vi "pumonarytesting_auto_attempt3.vi"() -> ()   [LabVIEW 2014]
uses:
  <vilib>/vision/NI_Vision_Development_Module.lvlib
  <instrlib>/KD Scientific 2XX Series/KD Scientific 2XX Series.lvlib
panel:
  in  "Number of Cycles":i32
  in  "Min Pressure":dbl
  in  "Max Pressure":dbl
  out "Status":T1
  in  "stop 2":bool
  out "Delivered Volume":dbl
  out "Units":string
  in  "Baud Rate (9600)":u32(ring)=9600 items=["300"=300, "1200"=1200, "2400"=2400, "4800"=4800, "9600"=9600]
  in  "Withdrawal Settings":T2={"Flow Rate (5)"=5.0, "Volume (10)"=10.0, "Volume Units (ml)"=enum."milliliters (ml)", "Rate Units (ml/min.)"=enum."milliliters per minute (ml/min.)"} {"Volume (10)" format="%#.3g"}
  in  "Diameter (8.75 mm)":dbl=8.75
  in  "Infusion Settings":T2={"Flow Rate (5)"=5.0, "Volume (10)"=10.0, "Volume Units (ml)"=enum."milliliters (ml)", "Rate Units (ml/min.)"=enum."milliliters per minute (ml/min.)"}
  in  "Address (0)":i32 format="%0.0f"
  in  "error in (no error)":errorcluster
  in  "VISA resource name":refnum<visa-resource-name>="COM1"
  in  "stop":bool
  out "Image":T3(plugin-control)
  out "Particle Measurements (Pixels) (Particle Analysis 1)":dbl[][](array[numeric]) format="%.2f"
  out "subarray":dbl[](array[numeric])
  out "The diameter":dbl[](array[numeric])
  in  "stop (F)":bool
  out "Data from Transducer":dynamicdata(graph) caption="Voltage from Transducer V"
  out "Voltage from pressure transducer":dbl[](array[numeric])
  out "Pressure mm Hg":dbl[](graph)
  in  "Calibration factor(-25.53)":dbl[](array[numeric])
  in  "Zero Error (-.09)":dbl[](array[numeric])
  out "pressure mm Hg":dbl[](array[numeric])
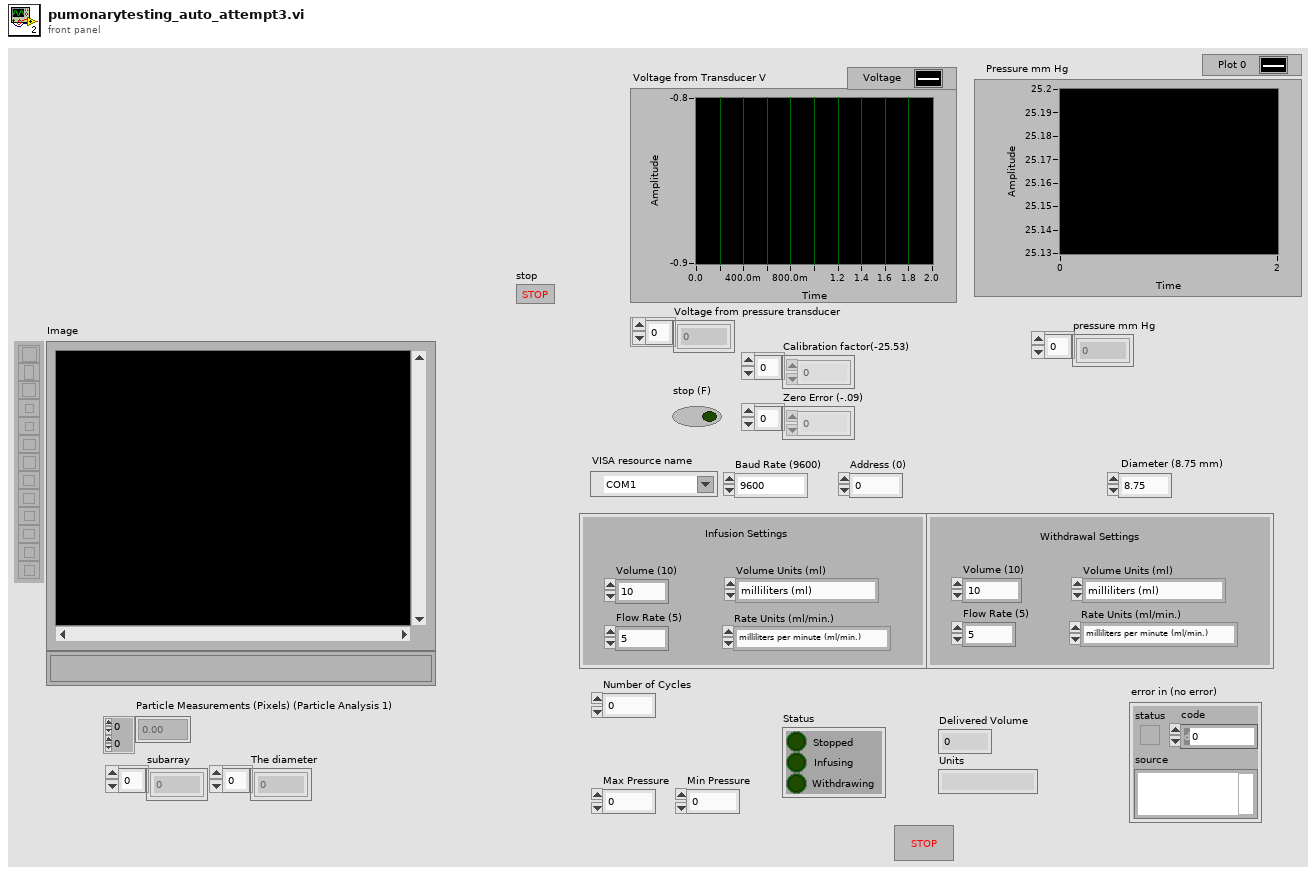
[diagram p1: front panel]
types:
  T1 = cluster{"Stopped":bool, "Infusing":bool, "Withdrawing":bool}
  T2 = cluster{"Flow Rate (5)":dbl, "Volume (10)":dbl, "Volume Units (ml)":enum16{"milliliters (ml)", "microliters (ul)"}, "Rate Units (ml/min.)":enum16{"milliliters per minute (ml/min.)", "milliliters per hour (ml/hr.)", "microliters per minute (ul/min.)", "microliters per hour (ul/hr.)"}}
  T3 = typedef "IMAQ Image.ctl" = refnum<image>
  T4 = typedef "Board Id" = u8
  T5 = typedef "ROI Descriptor" = cluster{"Global Rectangle":i32[], "Contours":cluster{"ID":enum32{"External", "Internal"}, "Type":u32, "Coordinates":i32[]}[]}
  T6 = enum16{"milliliters per minute (ml/min.)", "milliliters per hour (ml/hr.)", "microliters per minute (ul/min.)", "microliters per hour (ul/hr.)"}
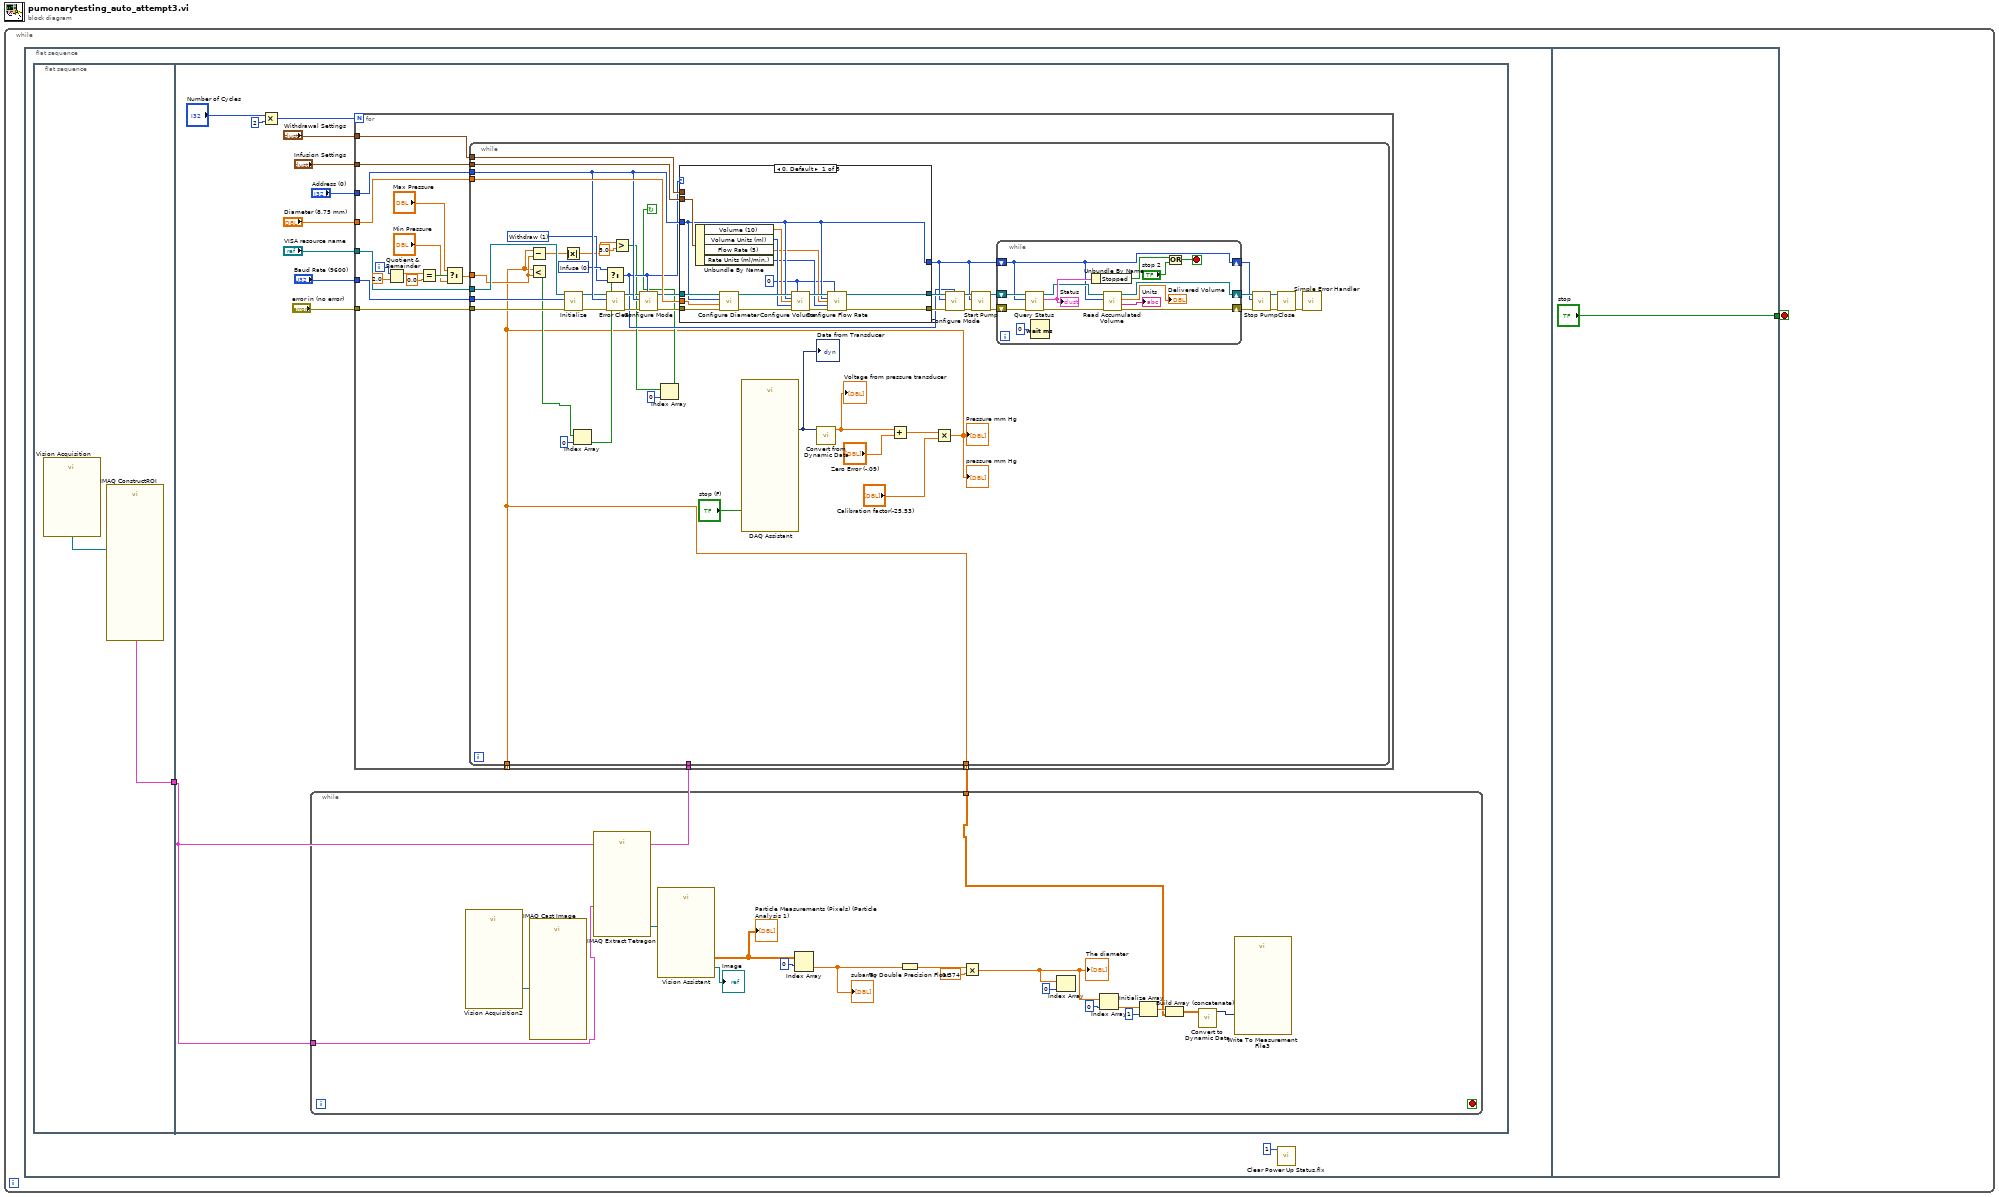
[diagram p0: block diagram]
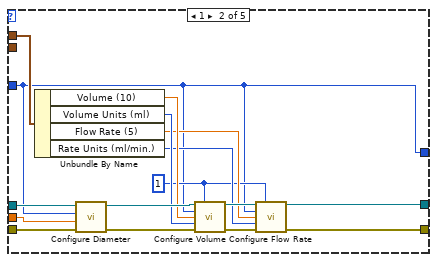
[diagram p2: hidden frame]
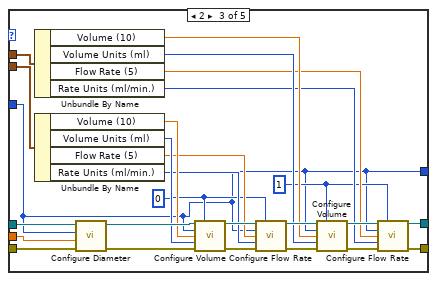
[diagram p3: hidden frame]
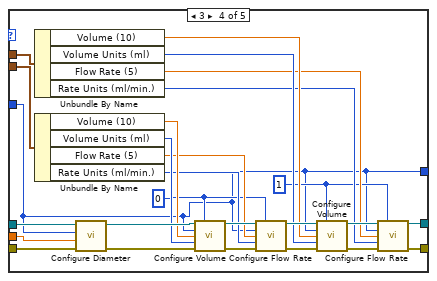
[diagram p4: hidden frame]
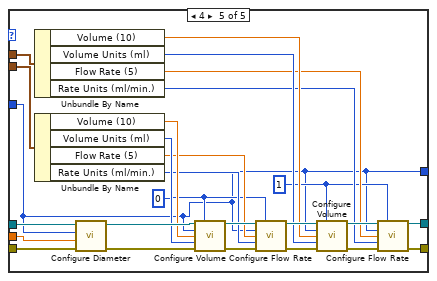
[diagram p5: hidden frame]
diagram:
  n1 = while {
    stop <- w1 stop-if-true
    n2 = flat-sequence {
      tunnel: ["stop"] -> w1
      frame #0 {
        n3 = flat-sequence {
          tunnel: [w4] -> w3
          tunnel: w3 -> [w6]
          frame #0 {
            n4 = call "Vision Acquisition"() -> ("Image Out"=w5:T3)  [unwired: 26 in, 1 out]
            n5 = call "IMAQ ConstructROI"("Image"=w5) -> ("ROI Descriptor Out"=w4:T5)  [unwired: 7 in, 3 out]
          }
          frame #1 {
            n6 = Multiply(x="Number of Cycles", y=2) -> (x*y=w17:i32)
            n7 = for {
              N: w17 -> [_]
              tunnel: "VISA resource name" -> [w53]
              tunnel: "error in (no error)" -> [w52]
              tunnel: "Infusion Settings" -> [w51]
              tunnel: "Withdrawal Settings" -> [w50]
              tunnel: "Diameter (8.75 mm)" -> [w49]
              tunnel: "Baud Rate (9600)" -> [w48]
              tunnel: "Address (0)" -> [w47]
              tunnel: [w38] -> _ mode=indexing
              tunnel: w6 -> [w37]
              tunnel: [w36] -> w7 mode=indexing
              i -> [w45]
              n8 = Quotient & Remainder(x=w45, y=2.0) -> (x-y*floor(x/y)=w43:dbl)  [unwired: 1 out]
              n9 = Equal?(x=w43, y=0.0) -> (x = y?=w42:bool)
              n10 = Select(t="Max Pressure", s=w42, f="Min Pressure") -> (s? t:f=w39:dbl)
              n11 = while {
                tunnel: w53 -> [w99]
                tunnel: w52 -> [w98]
                tunnel: w51 -> [w97]
                tunnel: w50 -> [w96]
                tunnel: w49 -> [w95]
                tunnel: w48 -> [w94]
                tunnel: w47 -> [w93]
                tunnel: w39 -> [w70]
                tunnel: [w54] -> w38
                tunnel: w37 -> [_]
                tunnel: [w54] -> w36
                stop <- w55 continue-if-true
                w72 = u16 1 items=["Withdraw"=1]
                w73 = u16 0 items=["Infuse"] ("Mode (infuse)")
                n12 = call <instrlib>:"Initialize.vi"("error in (no error)"=w98, "Baud Rate (9600)"=w94, "VISA resource name"=w99) -> ("error out"=w75:errorcluster, "VISA resource name out"=w74:refnum<visa-resource-name>)  [unwired: 7 in]
                n13 = call <instrlib>:"Error Clear.vi"("error in (no error)"=w75, "Address (0)"=w93, "VISA resource name"=w74) -> ("error out"=w76:errorcluster, "VISA resource name out"=w77:refnum<visa-resource-name>)  [unwired: 6 in, 1 out]
                n14 = call "DAQ Assistant"("stop (F)"="stop (F)") -> ("data"=w61:dynamicdata)  [unwired: 15 in, 3 out]
                "Data from Transducer" <- w61
                n15 = call "Convert from Dynamic Data"("Dynamic Data Type"=w61) -> ("Array"=w64:dbl[])  [unwired: 3 in]
                "Voltage from pressure transducer" <- w64
                n16 = Add(x=w64, y="Zero Error (-.09)") -> (x+y=w62:dbl[])
                n17 = Multiply(x=w62, y="Calibration factor(-25.53)") -> (x*y=w54:dbl[])
                "Pressure mm Hg" <- w54
                "pressure mm Hg" <- w54
                n18 = Subtract(x=w54, y=w70) -> (x-y=w69:dbl[])
                n19 = Less?(x=w54, y=w70) -> (x < y?=w60:bool[])
                n20 = Absolute Value(x=w69) -> (abs(x)=w68:dbl[])
                n21 = Index Array(array=w60, index=0) -> (element=w58:bool)
                n22 = Select(t=w73, s=w58, f=w72) -> (s? t:f=w71:u16)
                n23 = Greater?(x=w68, y=5.0) -> (0:w57:bool[])
                n24 = call <instrlib>:"Configure Mode.vi"("Mode (infuse)"=w71, "error in (no error)"=w76, "Address (0)"=w93, "VISA resource name"=w77) -> ("error out"=w79:errorcluster, "VISA resource name out"=w78:refnum<visa-resource-name>)  [unwired: 6 in]
                n25 = Index Array(array=w57, index=0) -> (element=w55:bool)
                n26 = case shown="0, Default" w71 {
                  tunnel: w97 -> [w109 _ w157 w183 w209]
                  tunnel: w96 -> [_ w131 w156 w182 w208]
                  tunnel: w78 -> [w115 w130 w155 w181 w207]
                  tunnel: w79 -> [w114 w126 w154 w180 w206]
                  tunnel: w95 -> [w108 w122 w137 w163 w189]
                  tunnel: [w107 w116 w132 w158 w184] -> w80
                  tunnel: w93 -> [w107 w116 w132 w158 w184]
                  tunnel: [w102 w127 w134 w160 w186] -> w84
                  tunnel: [w101 w123 w133 w159 w185] -> w83
                  frame 0, Default {
                    w100 = 0
                    n27 = Unbundle By Name(w109) -> ("Volume (10)"=w106:dbl, "Volume Units (ml)"=w105:enum16{"milliliters (ml)", "microliters (ul)"}, "Flow Rate (5)"=w104:dbl, "Rate Units (ml/min.)"=w103:T6)
                    n28 = call <instrlib>:"Configure Diameter.vi"("error in (no error)"=w114, "Diameter (8.75 mm)"=w108, "Address (0)"=w107, "VISA resource name"=w115) -> ("error out"=w112:errorcluster, "VISA resource name out"=w113:refnum<visa-resource-name>)  [unwired: 6 in]
                    n29 = call <instrlib>:"Configure Volume.vi"("VISA resource name"=w113, "Mode (infuse)"=w100, "Address (0)"=w107, "Volume (100)"=w106, "Units (0: milliliters)"=w105, "error in (no error)"=w112) -> ("VISA resource name out"=w111:refnum<visa-resource-name>, "error out"=w110:errorcluster)  [unwired: 8 in]
                    n30 = call <instrlib>:"Configure Flow Rate.vi"("VISA resource name"=w111, "Mode (infuse)"=w100, "Address (0)"=w107, "Flow Rate (5)"=w104, "Units (0: milliliters per minute)"=w103, "error in (no error)"=w110) -> ("VISA resource name out"=w102:refnum<visa-resource-name>, "error out"=w101:errorcluster)  [unwired: 8 in]
                  }
                  frame 1 {
                    w117 = 1
                    n31 = Unbundle By Name(w131) -> ("Volume (10)"=w121:dbl, "Volume Units (ml)"=w120:enum16{"milliliters (ml)", "microliters (ul)"}, "Flow Rate (5)"=w119:dbl, "Rate Units (ml/min.)"=w118:T6)
                    n32 = call <instrlib>:"Configure Diameter.vi"("error in (no error)"=w126, "Diameter (8.75 mm)"=w122, "Address (0)"=w116, "VISA resource name"=w130) -> ("error out"=w125:errorcluster, "VISA resource name out"=w129:refnum<visa-resource-name>)  [unwired: 6 in]
                    n33 = call <instrlib>:"Configure Volume.vi"("VISA resource name"=w129, "Mode (infuse)"=w117, "Address (0)"=w116, "Volume (100)"=w121, "Units (0: milliliters)"=w120, "error in (no error)"=w125) -> ("VISA resource name out"=w128:refnum<visa-resource-name>, "error out"=w124:errorcluster)  [unwired: 8 in]
                    n34 = call <instrlib>:"Configure Flow Rate.vi"("VISA resource name"=w128, "Mode (infuse)"=w117, "Address (0)"=w116, "Flow Rate (5)"=w119, "Units (0: milliliters per minute)"=w118, "error in (no error)"=w124) -> ("VISA resource name out"=w127:refnum<visa-resource-name>, "error out"=w123:errorcluster)  [unwired: 8 in]
                  }
                  frame 2 {
                    w135 = 1
                    w136 = 0
                    n35 = Unbundle By Name(w156) -> ("Volume (10)"=w141:dbl, "Volume Units (ml)"=w140:enum16{"milliliters (ml)", "microliters (ul)"}, "Flow Rate (5)"=w139:dbl, "Rate Units (ml/min.)"=w138:T6)
                    n36 = Unbundle By Name(w157) -> ("Volume (10)"=w145:dbl, "Volume Units (ml)"=w144:enum16{"milliliters (ml)", "microliters (ul)"}, "Flow Rate (5)"=w143:dbl, "Rate Units (ml/min.)"=w142:T6)
                    n37 = call <instrlib>:"Configure Diameter.vi"("error in (no error)"=w154, "Diameter (8.75 mm)"=w137, "Address (0)"=w132, "VISA resource name"=w155) -> ("error out"=w149:errorcluster, "VISA resource name out"=w153:refnum<visa-resource-name>)  [unwired: 6 in]
                    n38 = call <instrlib>:"Configure Volume.vi"("VISA resource name"=w153, "Mode (infuse)"=w136, "Address (0)"=w132, "Volume (100)"=w145, "Units (0: milliliters)"=w144, "error in (no error)"=w149) -> ("VISA resource name out"=w152:refnum<visa-resource-name>, "error out"=w148:errorcluster)  [unwired: 8 in]
                    n39 = call <instrlib>:"Configure Flow Rate.vi"("VISA resource name"=w152, "Mode (infuse)"=w136, "Address (0)"=w132, "Flow Rate (5)"=w143, "Units (0: milliliters per minute)"=w142, "error in (no error)"=w148) -> ("VISA resource name out"=w151:refnum<visa-resource-name>, "error out"=w147:errorcluster)  [unwired: 8 in]
                    n40 = call <instrlib>:"Configure Volume.vi"("VISA resource name"=w151, "Mode (infuse)"=w135, "Address (0)"=w132, "Volume (100)"=w141, "Units (0: milliliters)"=w140, "error in (no error)"=w147) -> ("VISA resource name out"=w150:refnum<visa-resource-name>, "error out"=w146:errorcluster)  [unwired: 8 in]
                    n41 = call <instrlib>:"Configure Flow Rate.vi"("VISA resource name"=w150, "Mode (infuse)"=w135, "Address (0)"=w132, "Flow Rate (5)"=w139, "Units (0: milliliters per minute)"=w138, "error in (no error)"=w146) -> ("VISA resource name out"=w134:refnum<visa-resource-name>, "error out"=w133:errorcluster)  [unwired: 8 in]
                  }
                  frame 3 {
                    w161 = 1
                    w162 = 0
                    n42 = Unbundle By Name(w182) -> ("Volume (10)"=w167:dbl, "Volume Units (ml)"=w166:enum16{"milliliters (ml)", "microliters (ul)"}, "Flow Rate (5)"=w165:dbl, "Rate Units (ml/min.)"=w164:T6)
                    n43 = Unbundle By Name(w183) -> ("Volume (10)"=w171:dbl, "Volume Units (ml)"=w170:enum16{"milliliters (ml)", "microliters (ul)"}, "Flow Rate (5)"=w169:dbl, "Rate Units (ml/min.)"=w168:T6)
                    n44 = call <instrlib>:"Configure Diameter.vi"("error in (no error)"=w180, "Diameter (8.75 mm)"=w163, "Address (0)"=w158, "VISA resource name"=w181) -> ("error out"=w175:errorcluster, "VISA resource name out"=w179:refnum<visa-resource-name>)  [unwired: 6 in]
                    n45 = call <instrlib>:"Configure Volume.vi"("VISA resource name"=w179, "Mode (infuse)"=w162, "Address (0)"=w158, "Volume (100)"=w171, "Units (0: milliliters)"=w170, "error in (no error)"=w175) -> ("VISA resource name out"=w178:refnum<visa-resource-name>, "error out"=w174:errorcluster)  [unwired: 8 in]
                    n46 = call <instrlib>:"Configure Flow Rate.vi"("VISA resource name"=w178, "Mode (infuse)"=w162, "Address (0)"=w158, "Flow Rate (5)"=w169, "Units (0: milliliters per minute)"=w168, "error in (no error)"=w174) -> ("VISA resource name out"=w177:refnum<visa-resource-name>, "error out"=w173:errorcluster)  [unwired: 8 in]
                    n47 = call <instrlib>:"Configure Volume.vi"("VISA resource name"=w177, "Mode (infuse)"=w161, "Address (0)"=w158, "Volume (100)"=w167, "Units (0: milliliters)"=w166, "error in (no error)"=w173) -> ("VISA resource name out"=w176:refnum<visa-resource-name>, "error out"=w172:errorcluster)  [unwired: 8 in]
                    n48 = call <instrlib>:"Configure Flow Rate.vi"("VISA resource name"=w176, "Mode (infuse)"=w161, "Address (0)"=w158, "Flow Rate (5)"=w165, "Units (0: milliliters per minute)"=w164, "error in (no error)"=w172) -> ("VISA resource name out"=w160:refnum<visa-resource-name>, "error out"=w159:errorcluster)  [unwired: 8 in]
                  }
                  frame 4 {
                    w187 = 1
                    w188 = 0
                    n49 = Unbundle By Name(w208) -> ("Volume (10)"=w193:dbl, "Volume Units (ml)"=w192:enum16{"milliliters (ml)", "microliters (ul)"}, "Flow Rate (5)"=w191:dbl, "Rate Units (ml/min.)"=w190:T6)
                    n50 = Unbundle By Name(w209) -> ("Volume (10)"=w197:dbl, "Volume Units (ml)"=w196:enum16{"milliliters (ml)", "microliters (ul)"}, "Flow Rate (5)"=w195:dbl, "Rate Units (ml/min.)"=w194:T6)
                    n51 = call <instrlib>:"Configure Diameter.vi"("error in (no error)"=w206, "Diameter (8.75 mm)"=w189, "Address (0)"=w184, "VISA resource name"=w207) -> ("error out"=w201:errorcluster, "VISA resource name out"=w205:refnum<visa-resource-name>)  [unwired: 6 in]
                    n52 = call <instrlib>:"Configure Volume.vi"("VISA resource name"=w205, "Mode (infuse)"=w188, "Address (0)"=w184, "Volume (100)"=w197, "Units (0: milliliters)"=w196, "error in (no error)"=w201) -> ("VISA resource name out"=w204:refnum<visa-resource-name>, "error out"=w200:errorcluster)  [unwired: 8 in]
                    n53 = call <instrlib>:"Configure Flow Rate.vi"("VISA resource name"=w204, "Mode (infuse)"=w188, "Address (0)"=w184, "Flow Rate (5)"=w195, "Units (0: milliliters per minute)"=w194, "error in (no error)"=w200) -> ("VISA resource name out"=w203:refnum<visa-resource-name>, "error out"=w199:errorcluster)  [unwired: 8 in]
                    n54 = call <instrlib>:"Configure Volume.vi"("VISA resource name"=w203, "Mode (infuse)"=w187, "Address (0)"=w184, "Volume (100)"=w193, "Units (0: milliliters)"=w192, "error in (no error)"=w199) -> ("VISA resource name out"=w202:refnum<visa-resource-name>, "error out"=w198:errorcluster)  [unwired: 8 in]
                    n55 = call <instrlib>:"Configure Flow Rate.vi"("VISA resource name"=w202, "Mode (infuse)"=w187, "Address (0)"=w184, "Flow Rate (5)"=w191, "Units (0: milliliters per minute)"=w190, "error in (no error)"=w198) -> ("VISA resource name out"=w186:refnum<visa-resource-name>, "error out"=w185:errorcluster)  [unwired: 8 in]
                  }
                }
                n56 = call <instrlib>:"Configure Mode.vi"("Mode (infuse)"=w71, "error in (no error)"=w83, "Address (0)"=w80, "VISA resource name"=w84) -> ("error out"=w81:errorcluster, "VISA resource name out"=w82:refnum<visa-resource-name>)  [unwired: 6 in]
                n57 = call <instrlib>:"Start Pump.vi"("error in (no error)"=w81, "Address (0)"=w80, "VISA resource name"=w82) -> ("error out"=w91:errorcluster, "VISA resource name out"=w92:refnum<visa-resource-name>)  [unwired: 7 in]
                n58 = while {
                  shift-right: [w212] -> w88
                  shift-left: w80 -> [w212]
                  shift-right: [w214] -> w90
                  shift-left: w92 -> [w220]
                  shift-right: [w213] -> w89
                  shift-left: w91 -> [w221]
                  stop <- w218 stop-if-true
                  n59 = call <instrlib>:"Query Status.vi"("error in (no error)"=w221, "Address (0)"=w212, "VISA resource name"=w220) -> ("error out"=w223:errorcluster, "Status"=w219:T1, "VISA resource name out"=w215:refnum<visa-resource-name>)  [unwired: 6 in]
                  "Status" <- w219
                  n60 = Wait (ms)(milliseconds to wait=u32 0) -> ()  [unwired: 1 out]
                  n61 = Unbundle By Name(w219) -> ("Stopped"=w217:bool)
                  n62 = call <instrlib>:"Read Accumulated Volume.vi"("error in (no error)"=w223, "Address (0)"=w212, "VISA resource name"=w215) -> ("error out"=w213:errorcluster, "Units"=→"Units":string, "Delivered Volume"=→"Delivered Volume":dbl, "VISA resource name out"=w214:refnum<visa-resource-name>)  [unwired: 5 in]
                  n63 = Or(x=w217, y="stop 2") -> (x .or. y?=w218:bool)
                }
                n64 = call <instrlib>:"Stop Pump.vi"("error in (no error)"=w89, "Address (0)"=w88, "VISA resource name"=w90) -> ("error out"=w86:errorcluster, "VISA resource name out"=w85:refnum<visa-resource-name>)  [unwired: 7 in]
                n65 = call <instrlib>:"Close.vi"("error in (no error)"=w86, "VISA resource name"=w85) -> ("error out"=w87:errorcluster)  [unwired: 9 in]
                n66 = call <vilib>:"Simple Error Handler.vi"("error in (no error)"=w87) -> ()  [unwired: 4 in, 5 out]
              }
            }
            n67 = while {
              tunnel: w7 -> [w19]
              tunnel: w6 -> [w18]
              stop <- _ stop-if-true
              n68 = call "Vision Acquisition2"() -> ("Image Out"=w27:T3)  [unwired: 25 in, 2 out]
              n69 = call "IMAQ Cast Image"("Image Src"=w27) -> ()  [unwired: 9 in, 2 out]
              n70 = call-poly "IMAQ Extract Tetragon"("ROI Descriptor"=w18) -> ("Image Dst Out"=w34:T3)  [unwired: 9 in, 1 out]
              n71 = call "Vision Assistant"("Image In"=w34) -> ("Image Out"=→"Image":T3, "Particle Measurements (Pixels) (Particle Analysis 1)"=w33:dbl[][])  [unwired: 23 in, 2 out]
              "Particle Measurements (Pixels) (Particle Analysis 1)" <- w33
              n72 = Index Array(array=w33, index (row)=0) -> (element=w31:dbl[])  [unwired: 1 in]
              "subarray" <- w31
              n73 = To Double Precision Float(number=w31) -> (double precision float=w30:dbl[])
              n74 = Multiply(x=w30, y=0.374) -> (x*y=w25:dbl[])
              "The diameter" <- w25
              n75 = Index Array(array=w25, index=0) -> ()  [unwired: 1 out]
              n76 = Index Array(array=w25, index=0) -> (element=w24:dbl)
              n77 = Initialize Array(w24, 1 ("dimension size")) -> (w22:dbl[])
              n78 = Build Array (concatenate)(w22, w19) -> (w21:dbl[][])
              n79 = call "Convert to Dynamic Data"("2D Array"=w21) -> ("Dynamic Data Type"=w20:dynamicdata)  [unwired: 3 in]
              n80 = call "Write To Measurement File3"("Signals"=w20) -> ()  [unwired: 16 in, 3 out]
            }
          }
        }
        n81 = call <vilib>:"Clear Power Up Status.flx"("Board ID"=T4 1) -> ()  [unwired: 6 in, 2 out]
      }
      frame #1 {
      }
    }
  }
